vi "fpga_sysID_Z_axis.vi"() -> ()   [LabVIEW 2017]
uses:
  controls/boolean_info.ctl
  sysID_Z-axis-params.ctl
  <vilib>/rvi/Emulation/niFpgaGetClockAttributes.vi
  <vilib>/rvi/Emulation/niFpgaSctlEmulationGetInTimedLoop.vi
  <vilib>/rvi/Emulation/niFpgaEmulationReportErrorSimple.vi
  <vilib>/rvi/Emulation/niFpgaProcessEmulError.vi
  <vilib>/rvi/eio/common/nirviEmuTemplateMethod_errors.vi
  <vilib>/rvi/Emulation/niFpgaEmulationIsFPGAContextNoSignature.vi
  <vilib>/rvi/DataTransferAndStorage/Container/Common/niFpgaContainerGetUniqueNameForEmu.vi
  <vilib>/rvi/Memory/Memory_Emulation/niFpgaMemoryEmulationCacheClearOnFirstRun.vi
  <vilib>/rvi/Memory/Memory_Emulation/nirvimemoryEmulationManagerCache_MakeExclusive.vi
  <vilib>/rvi/Memory/Memory_Emulation/niFpgaMemoryEmulationValidateCache.vi
  <vilib>/rvi/Memory/Memory_Emulation/nirvimemoryEmulationManagerCache_InsertValue.vi
  <vilib>/Utility/error.llb/Clear Errors.vi
  <vilib>/rvi/Memory/Memory_Emulation/nirvimemoryEmulationManagerCache_ReleaseExclusive.vi
  <vilib>/rvi/Memory/Memory_Emulation/nirvimemoryEmulationManagerCache_GetValue.vi
  <vilib>/rvi/Memory/Memory_Emulation/nirvimemoryEmulationManagerCache_SetValue.vi
  <vilib>/rvi/Emulation/niFpgaCriticalErrorInLSC.vi
  <vilib>/eio/EIONode/EIONode.xnode
  <vilib>/rvi/DataTransferAndStorage/Container/XNode/niFpgaContainer.xnode
  <vilib>/rvi/DataTransferAndStorage/Register/Emulation/niFpgaRegisterEmulation.vi
  FPGA-data-logging.lvlib
  libimaging-cs.lvlib
panel:
  in  "sysID_Z_axis_params":T1={"TOL"=0.3, "ramp-rate"=-5e-06, "z-u-max"=5.0, "offset"=0.0, "Ki"=0.001, "Z-error-threshold"=0.0, "Z-settled-samples\nthreshold "=0, "z_UP"=1.5, "zup-N"=5000} {"Z-error-threshold" format="%#_13g"; "ramp-rate" format="%#_4g"; "TOL" format="%#_13g"}
  out "iter":i32
  out "freqIndex":i16
  out "All Done":bool
  in  "TsTicks":u32=1600
  out "Current Case":i16
  out "boolean \nindicators":T2
  out "z-u(k)":sgl
  in  "ABORT":bool
  out "read fifo HARD timeout":bool
  in  "numFreqs":i16
  out "e(0) (threshhold init)":fxp<+/-,16,5>
  in  "init Z up":fxp<+/-,16,5>
  in  "trigger-0":bool
  in  "initial case":i16
  # "- If collect all = fasle and collect move = false,\nwe only collect measurement data.\n- If collect all = false, and collect move = true,\nwe collect measurement and move data.\n- If collect all = true, we collect everything."
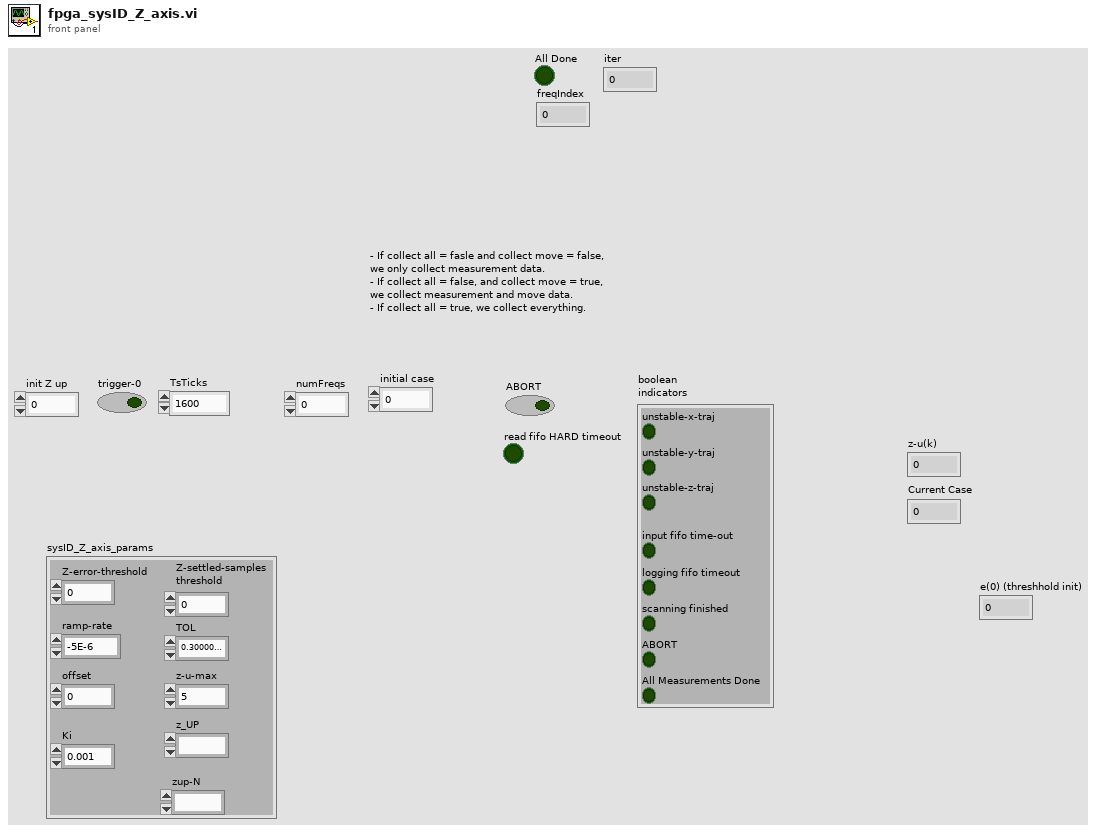
[diagram p1: front panel]
types:
  T1 = typedef "sysID_Z-axis-params.ctl" = cluster{"TOL":sgl, "ramp-rate":sgl, "z-u-max":sgl, "offset":sgl, "Ki":sgl, "Z-error-threshold":sgl, "Z-settled-samples\nthreshold ":i16, "z_UP":fxp<+/-,16,5>, "zup-N":i16}
  T2 = typedef "boolean_info.ctl" = cluster{"unstable-z-traj":bool, "input fifo time-out":bool, "logging fifo timeout":bool, "scanning finished":bool, "unstable-x-traj":bool, "unstable-y-traj":bool, "ABORT":bool, "All Measurements Done":bool}
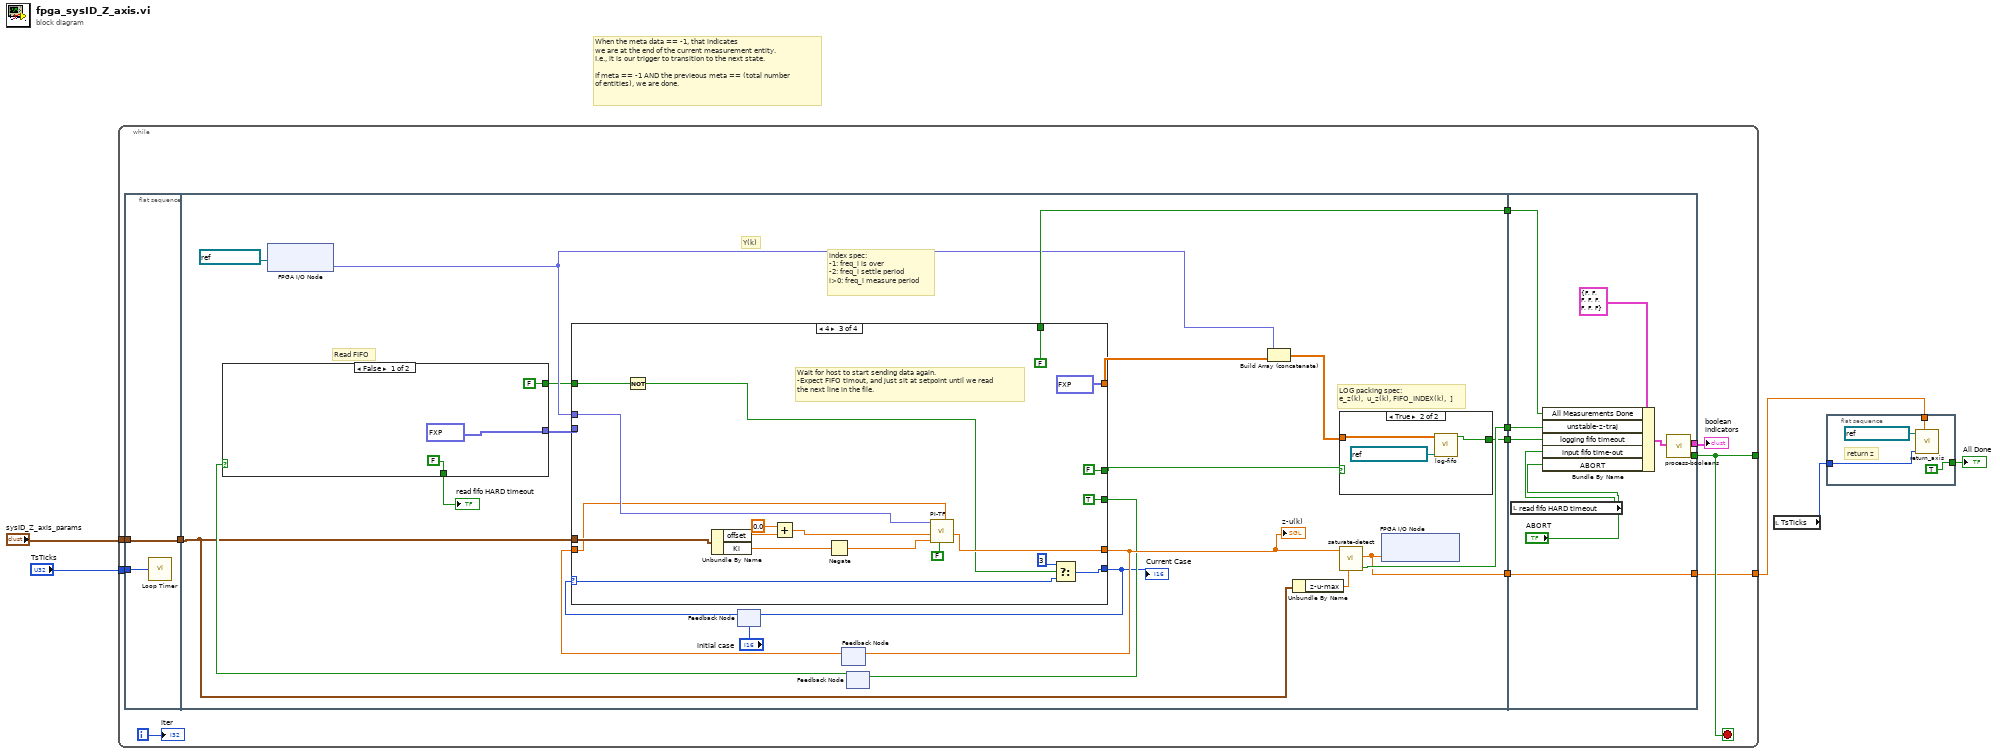
[diagram p0: block diagram]
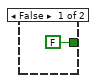
[diagram p2: hidden frame]
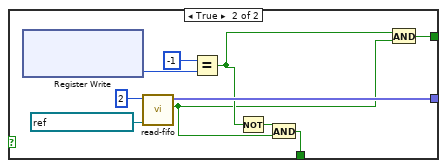
[diagram p3: hidden frame]
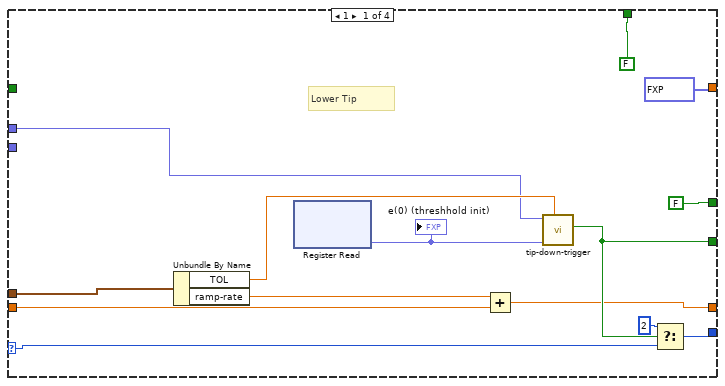
[diagram p4: hidden frame]
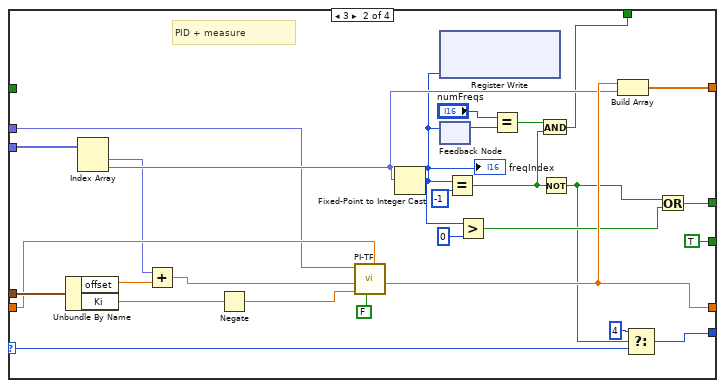
[diagram p5: hidden frame]
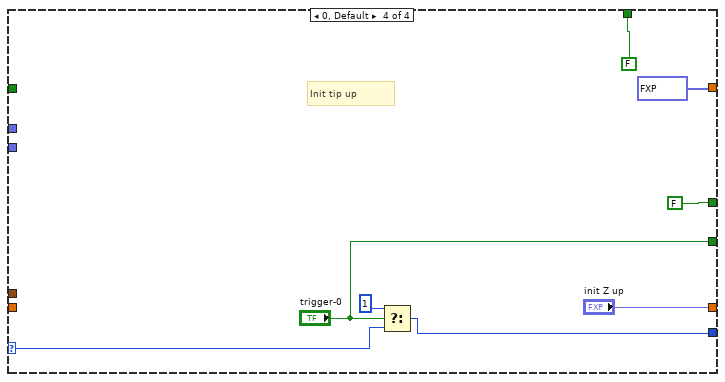
[diagram p6: hidden frame]
diagram:
  # "When the meta data == -1, that indicates\nwe are at the end of the current measurement entity.\nI.e., it is our trigger to transition to the next state.\n\nIf meta == -1 AND the previeous meta == (total number\nof entities), we are done."
  n1 = while {
    tunnel: "sysID_Z_axis_params" -> [w12]
    tunnel: "TsTicks" -> [w11]
    tunnel: [w9] -> _
    tunnel: [w7] -> w4
    i -> [w6]
    stop <- w9 stop-if-true
    n2 = flat-sequence {
      tunnel: w11 -> [w17]
      tunnel: w12 -> [w18]
      tunnel: [w18] -> w16
      tunnel: w16 -> [w27]
      tunnel: [w34] -> w15
      tunnel: [w33] -> w14
      tunnel: [w25] -> w13
      tunnel: [w29] -> w8
      tunnel: w15 -> [w135]
      tunnel: w14 -> [w132]
      tunnel: w13 -> [w129]
      tunnel: [w128] -> w9
      tunnel: [w127] -> w10
      tunnel: [w126] -> w7
      tunnel: w8 -> [w126]
      frame #0 {
        n3 = call "Loop Timer"("Count(Ticks)"=w17) -> ()  [unwired: 1 out]
      }
      frame #1 {
        # "index spec:\n-1: freq_i is over\n-2: freq_i settle period\ni>0: freq_i measure period"
        # "Y(k)"
        # "LOG packing spec:\ne_z(k),  u_z(k), FIFO_INDEX(k),  ]"
        # "Read FIFO"
        n4 = xnode "FPGA I/O Node"("FPGA I/O In"=refnum<k21> "Mod2/AI2" ("y - ADC")) -> ("I/O Item"=w20:fxp<+/-,24,5>)  [unwired: 1 out]
        n5 = feedback #1("initial case") -> (w38:i16)
        n6 = feedback #2() -> (w37:sgl)  [unwired: 1 in]
        n7 = feedback #3() -> (w30:bool)  [unwired: 1 in]
        n8 = case shown="False" w30 {
          tunnel: [fxp<+/-,16,5>[] [0.0, 0.0] ("unpacked-data") w54] -> w28
          tunnel: [FALSE ("timout?") w47] -> w32
          tunnel: [FALSE w51] -> w19
          frame False {
          }
          frame True {
            n9 = xnode "Register Write"() -> ("Data"=w53:i16)  [unwired: 1 in, 1 out]
            n10 = call "read-fifo.vi"("FIFO In"=refnum<k21> "Host_to_FPGA", "numChan"=2) -> ("timout?"=w48:bool, "unpacked-data"=w54:fxp<+/-,16,5>[])  [unwired: 8 in]
            n11 = Equal?(x=i16 -1, y=w53) -> (x = y?=w49:bool)
            n12 = Not(x=w49) -> (.not. x?=w50:bool)
            n13 = And(x=w50, y=w48) -> (x .and. y?=w47:bool)
            n14 = And(x=w49, y=w48) -> (x .and. y?=w51:bool)
          }
        }
        "read fifo HARD timeout" <- w32
        n15 = case shown="4" w38 {
          selector: w38 -> [w67 w73 w104 w123]
          tunnel: [FALSE w79 FALSE FALSE] -> w22
          tunnel: [w65 w74 w105 w125] -> w23
          tunnel: w20 -> [w57 w76 w111 _]
          tunnel: [w60 TRUE ("trigger-0") TRUE ("trigger-0") "trigger-0"] -> w31
          tunnel: [w59 w89 w109 "init Z up"] -> w36
          tunnel: w37 -> [w63 w93 w110 _]
          tunnel: w27 -> [w66 w95 w112 _]
          tunnel: w28 -> [_ w88 _ _]
          tunnel: [FALSE w86 FALSE FALSE] -> w25
          tunnel: [fxp<+/-,16,5>[] [0.0, 0.0] ("unpacked-data") w84 fxp<+/-,16,5>[] [0.0, 0.0] ("unpacked-data") fxp<+/-,16,5>[] [0.0, 0.0] ("unpacked-data")] -> w24
          tunnel: w19 -> [_ _ w101 _]
          frame 1 {
            # "Lower Tip"
            n16 = Unbundle By Name(w66) -> ("TOL"=w69:sgl, "ramp-rate"=w68:sgl)
            n17 = xnode ("Register Read")() -> ("Data"=w70:fxp<+/-,16,5>)  [unwired: 1 in, 1 out]
            "e(0) (threshhold init)" <- w70
            n18 = Add(x=w68, y=w63) -> (x+y=w59:sgl)
            n19 = call "tip-down-trigger.vi"("TOL"=w69, "Vo"=w70, "e(k)"=w57) -> ("trigger"=w60:bool)  [unwired: 8 in]
            n20 = Select(t=i16 2, s=w60, f=w67) -> (s? t:f=w65:i16)
          }
          frame 3 {
            # "PID + measure"
            n21 = Unbundle By Name(w95) -> ("offset"=w81:sgl, "Ki"=w96:sgl)
            n22 = Index Array(array=w88) -> (element #1=w82:fxp<+/-,16,5>, element #2=w87:fxp<+/-,16,5>)  [unwired: 2 in]
            n23 = Add(x=w82, y=w81) -> (x+y=w83:sgl)
            n24 = Negate(x=w96) -> (-x=w97:sgl)
            n25 = call "PI-TF.vi"("u(k-1)"=w93, "reset"=FALSE, "Ki"=w97, "setpoint"=w83, "y(k)"=w76) -> ("u(k)"=w89:sgl)  [unwired: 6 in]
            n26 = Fixed-Point to Integer Cast(1:w87) -> (0:w71:i16)
            "freqIndex" <- w71
            n27 = xnode "Register Write"("Data"=w71) -> ()  [unwired: 1 in, 1 out]
            n28 = feedback #4() -> (w90:i16)  [unwired: 1 in]
            n29 = feedback-in #4(w71) -> ()
            n30 = Equal?(x=w71, y=i16 -1) -> (x = y?=w85:bool)
            n31 = Greater?(x=w71, y=i16 0) -> (0:w78:bool)
            n32 = Equal?(x="numFreqs", y=w90) -> (x = y?=w91:bool)
            n33 = And(x=w91, y=w85) -> (x .and. y?=w86:bool)
            n34 = Not(x=w85) -> (.not. x?=w72:bool)
            n35 = Build Array(w89, w87) -> (w84:sgl[])
            n36 = Select(t=i16 4, s=w72, f=w73) -> (s? t:f=w74:i16)
            n37 = Or(x=w72, y=w78) -> (x .or. y?=w79:bool)
          }
          frame 4 {
            # "Wait for host to start sending data again.\n-Expect FIFO timout, and just sit at setpoint until we read\nthe next line in the file."
            n38 = Not(x=w101) -> (.not. x?=w100:bool)
            n39 = Unbundle By Name(w112) -> ("offset"=w113:sgl, "Ki"=w115:sgl)
            n40 = Add(x=sgl 0.0, y=w113) -> (x+y=w114:sgl)
            n41 = Negate(x=w115) -> (-x=w116:sgl)
            n42 = call "PI-TF.vi"("u(k-1)"=w110, "reset"=FALSE, "Ki"=w116, "setpoint"=w114, "y(k)"=w111) -> ("u(k)"=w109:sgl)  [unwired: 6 in]
            n43 = Select(t=i16 3, s=w100, f=w104) -> (s? t:f=w105:i16)
          }
          frame 0, Default {
            # "Init tip up"
            n44 = Select(t=i16 1, s="trigger-0", f=w123) -> (s? t:f=w125:i16)
          }
        }
        "z-u(k)" <- w36
        "Current Case" <- w23
        n45 = feedback-in #1(w23) -> ()
        n46 = feedback-in #2(w36) -> ()
        n47 = feedback-in #3(w31) -> ()
        n48 = Build Array (concatenate)(w20, w24) -> (w35:sgl[])
        n49 = Unbundle By Name(w27) -> ("z-u-max"=w26:sgl)
        n50 = case shown="True" w22 {
          tunnel: w35 -> [_ w42]
          tunnel: [FALSE ("logging-timeout?") w41] -> w33
          frame False {
          }
          frame True {
            n51 = call "log-fifo.vi"("FIFO In"=refnum<k21> "fpga-to-host2", "input-data"=w42) -> ("logging-timeout?"=w41:bool)  [unwired: 9 in]
          }
        }
        n52 = call "saturate-detect.vi"("bound"=w26, "x"=w36) -> ("saturated"=w34:bool, "sat(x)"=w29:sgl)  [unwired: 8 in]
        n53 = xnode "FPGA I/O Node"("Mod1/AO2"=w29) -> ()  [unwired: 1 in, 1 out]
      }
      frame #2 {
        n54 = local read "read fifo HARD timeout"() -> (w131:bool)
        n55 = Bundle By Name(cluster=T2 {"unstable-z-traj"=FALSE, "input fifo time-out"=FALSE, "logging fifo timeout"=FALSE, "scanning finished"=FALSE, "unstable-x-traj"=FALSE, "unstable-y-traj"=FALSE, "ABORT"=FALSE, "All Measurements Done"=FALSE} ("boolean errors"), "All Measurements Done"=w129, "unstable-z-traj"=w135, "logging fifo timeout"=w132, "input fifo time-out"=w131, "ABORT"="ABORT") -> (w133:T2)
        n56 = call "process-booleans.vi"("boolean indicators 2"=w133) -> ("scaning finished"=w128:bool, "boolean indicators"=w127:T2)  [unwired: 9 in]
      }
    }
    "boolean \nindicators" <- w10
    "iter" <- w6
  }
  n57 = local read "TsTicks"() -> (w1:u32)
  n58 = flat-sequence {
    tunnel: w4 -> [w139]
    tunnel: [TRUE] -> w3
    tunnel: w1 -> [w136]
    frame #0 {
      # "return z"
      n59 = call "return_axis.vi"("u(0)"=w139, "TsTicks"=w136, "FPGA I/O In"=refnum<k21> "Mod1/AO2") -> ()  [unwired: 9 in]
    }
  }
  "All Done" <- w3
